vi "MIU_Control_v1.0 (2).vi"() -> ()   [LabVIEW 2010]
uses:
  <vilib>/Instr/_visa.llb/VISA Configure Serial Port (Instr).vi
  <vilib>/Analysis/NI_AALPro.lvlib
panel:
  in  "Tab Control":T1(tab)
  in  "Intrument Serial Input":refnum<visa-resource-name>="COM4"
  in  "data bits":u16=8 min=5 max=8 step=1
  in  "parity":u16(ring) items=["None", "Odd", "Even", "Mark", "Space"]
  in  "stop bits":u16(ring)=10 items=["1.0"=10, "1.5"=15, "2.0"=20]
  in  "flow control":u16(ring) items=["None"=0, "XON/XOFF"=1, "RTS/CTS"=2, "DTR/DSR"=4]
  in  "delay before read (ms)":u32=500
  in  "byte count":u32=500
  out "Incoming Serial String":string
  out "Time":string
  out "Date":string
  in  "stop":bool
  in  "Control Unit Port":refnum<visa-resource-name>="COM4"
  in  "baud rate (9600)":u32=9600
  in  "baud rate (9600)":u32=9600
  out "N2O is FLAT":bool
  out "Rolling CO Slope Fit":cluster{i32[], "Best Linear Fit":dbl[]}[](graph)
  out "CO":dbl(graph)=0.310407
  out "N2O":dbl(graph)
  out "H2O":dbl(graph)
  out "CO PPM":string
  out "N2O PPM":string
  out "H2O PPM":string
  out "CO DRY":dbl(graph)
  out "CO DRY":string
  out "N2O DRY 2":string
  out "N2O DRY":dbl(graph)
  in  "Average Points":i32
  out "slope":dbl
  out "Rolling N2O Slope Fit 2":cluster{i32[], "Best Linear Fit":dbl[]}[](graph)
  out "slope 2":dbl
  in  "N2O Low Limit":dbl
  in  "CO High Limit":dbl
  out "CO is FLAT":bool
  in  "CO Low Limit":dbl
  in  "N2O High Limit":dbl
  out "CELL TEMP":string
  out "CELL TEMPERATURE":dbl(graph)
  out "AMBIENT TEMPERATURE":dbl(graph)
  out "AMBIENT TEMP":string
  out "AIN5":dbl(graph)
  out "SUPERCOOL TEMP":string
  out "LINE LOCK":dbl(graph)
  out "LINELOCK - LASER CONTROL VOLTAGE":string
  out "PRESSURE":dbl(graph)
  out "PRESSURE 2":string
  out "SuperCool Temperature":dbl
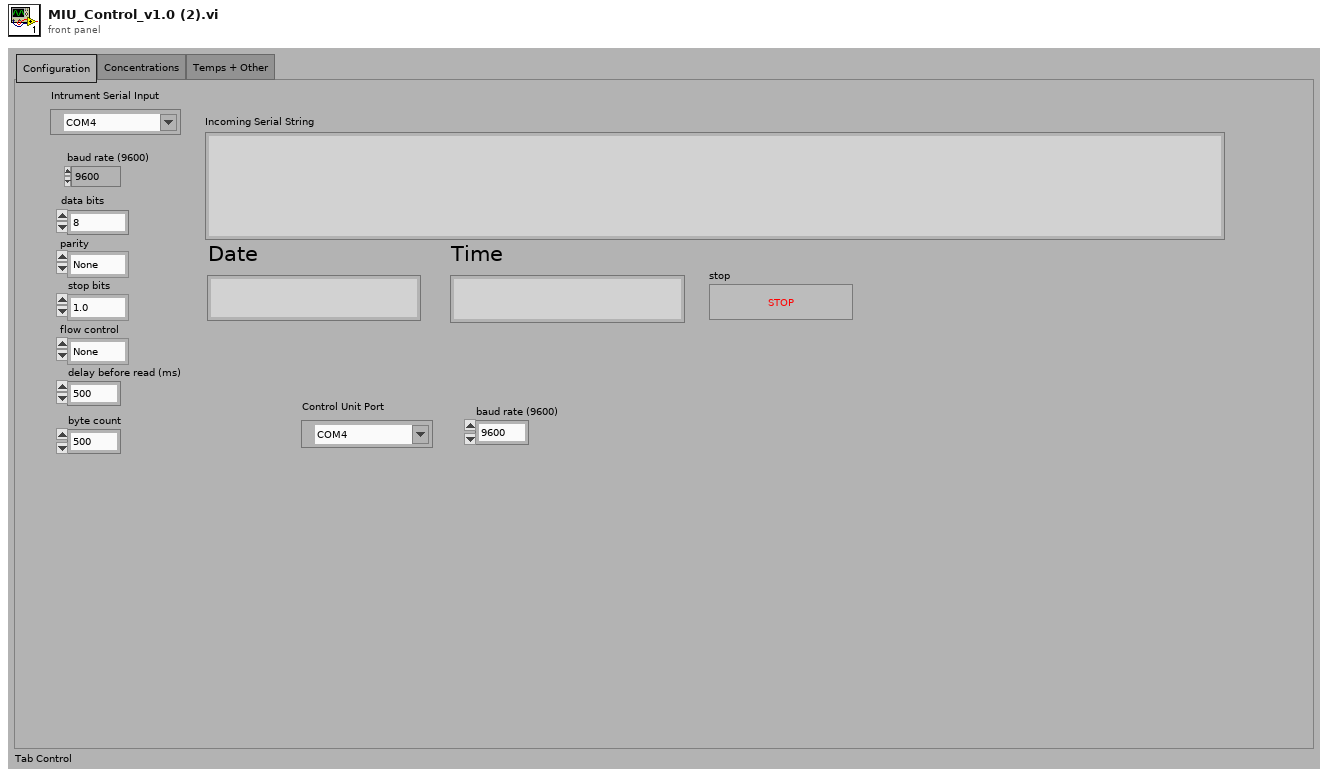
[diagram p1: front panel]
types:
  T1 = enum32{"Configuration", "Concentrations", "Temps + Other"}
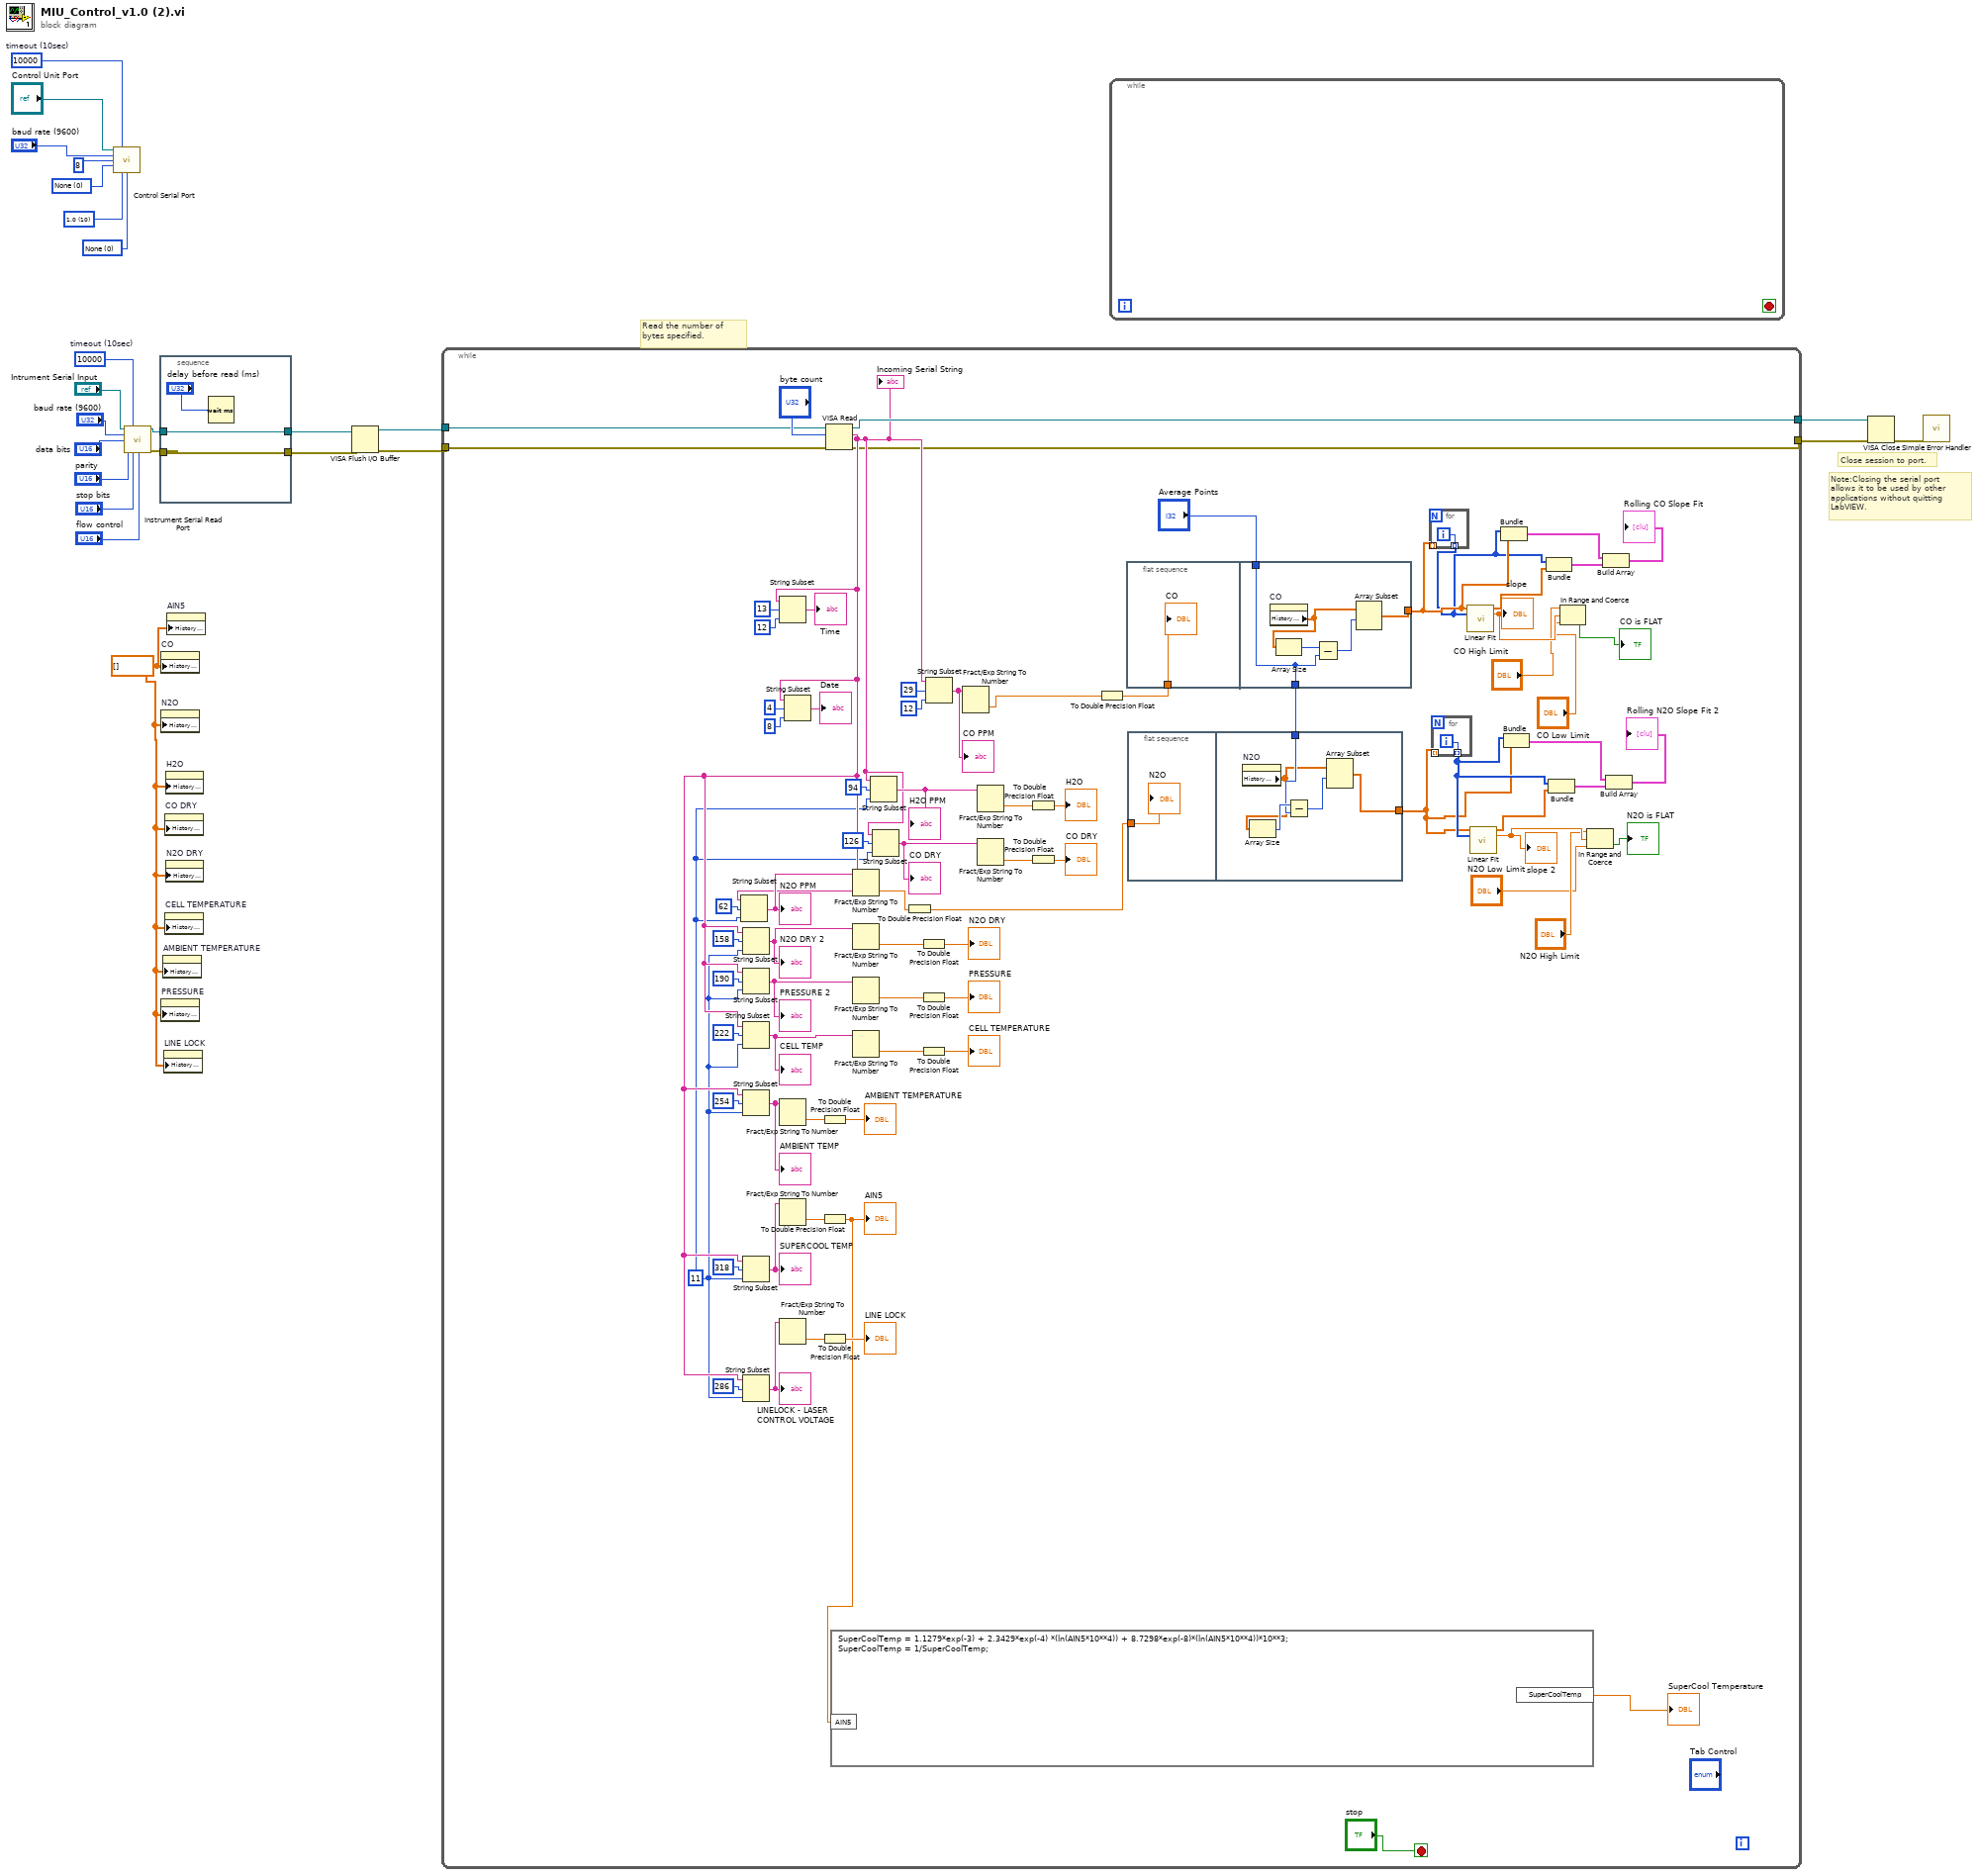
[diagram p0: block diagram]
diagram:
  w3 = u16 0 items=["None"=0, "XON/XOFF"=1, "RTS/CTS"=2, "DTR/DSR"=4] ("flow control")
  w4 = u16 10 items=["1.0"=10, "1.5"=15, "2.0"=20] ("stop bits")
  w6 = u16 0 items=["None", "Odd", "Even", "Mark", "Space"] ("parity")
  w5 = u32 10000  # timeout (10sec)
  w9 = dbl[] [] ("History Data")
  w21 = u32 10000  # timeout (10sec)
  # "Read the number of bytes specified."
  # "Note:Closing the serial port allows it to be used by other applications without quitting LabVIEW."
  # "Close session to port."
  n1 = call-poly "Control Serial Port"("VISA resource name"="Control Unit Port", "timeout (10sec)"=w5, "baud rate (9600)"="baud rate (9600)", "data bits (8)"=u16 8 ("data bits"), "parity (0:none)"=w6, "stop bits (10: 1 bit)"=w4, "flow control (0:none)"=w3) -> ()  [unwired: 2 in, 7 out]
  n2 = call-poly "Instrument Serial Read Port"("VISA resource name"="Intrument Serial Input", "timeout (10sec)"=w21, "baud rate (9600)"="baud rate (9600)", "data bits (8)"="data bits", "parity (0:none)"="parity", "stop bits (10: 1 bit)"="stop bits", "flow control (0:none)"="flow control") -> ("VISA resource name out"=w16:refnum<visa-resource-name>, "error out"=w17:errorcluster)  [unwired: 2 in, 5 out]
  n3 = stacked-sequence {
    tunnel: w17 -> [w27]
    tunnel: [w27] -> w10
    tunnel: w16 -> [w26]
    tunnel: [w26] -> w11
    frame #0 {
      n4 = Wait (ms)(milliseconds to wait="delay before read (ms)") -> ()  [unwired: 1 out]
    }
  }
  n5 = property on="CO" class="WFChart (strict)"("History Data"=w9) -> ()  [unwired: 2 in, 2 out]
  n6 = property on="N2O" class="WFChart (strict)"("History Data"=w9) -> ()  [unwired: 2 in, 2 out]
  n7 = property on="PRESSURE" class="WFChart (strict)"("History Data"=w9) -> ()  [unwired: 2 in, 2 out]
  n8 = property on="AMBIENT TEMPERATURE" class="WFChart (strict)"("History Data"=w9) -> ()  [unwired: 2 in, 2 out]
  n9 = property on="LINE LOCK" class="WFChart (strict)"("History Data"=w9) -> ()  [unwired: 2 in, 2 out]
  n10 = property on="CO DRY" class="WFChart (strict)"("History Data"=w9) -> ()  [unwired: 2 in, 2 out]
  n11 = property on="CELL TEMPERATURE" class="WFChart (strict)"("History Data"=w9) -> ()  [unwired: 2 in, 2 out]
  n12 = property on="H2O" class="WFChart (strict)"("History Data"=w9) -> ()  [unwired: 2 in, 2 out]
  n13 = property on="N2O DRY" class="WFChart (strict)"("History Data"=w9) -> ()  [unwired: 2 in, 2 out]
  n14 = property on="AIN5" class="WFChart (strict)"("History Data"=w9) -> ()  [unwired: 2 in, 2 out]
  n15 = VISA Flush I/O Buffer(VISA resource name=w11, error in (no error)=w10) -> (VISA resource name out=w13:refnum<visa-resource-name>, error out=w12:errorcluster)  [unwired: 1 in]
  n16 = while {
    tunnel: w13 -> [w74]
    tunnel: w12 -> [w75]
    tunnel: [w98] -> w15
    tunnel: [w53] -> w14
    stop <- "stop" stop-if-true
    w64 = 11 ("offset (0)")
    n17 = VISA Read(VISA resource name=w74, byte count="byte count", error in (no error)=w75) -> (VISA resource name out=w98:refnum<visa-resource-name>, read buffer=w65:string, error out=w53:errorcluster)  [unwired: 1 out]
    "Incoming Serial String" <- w65
    n18 = String Subset(string=w65, offset (0)=62, length (rest)=w64) -> (substring=w91:string)
    "N2O PPM" <- w91
    n19 = String Subset(string=w65, offset (0)=158, length (rest)=w64) -> (substring=w78:string)
    "N2O DRY 2" <- w78
    n20 = String Subset(string=w65, offset (0)=190, length (rest)=w64) -> (substring=w77:string)
    "PRESSURE 2" <- w77
    n21 = String Subset(string=w65, offset (0)=222, length (rest)=w64) -> (substring=w76:string)
    "CELL TEMP" <- w76
    n22 = String Subset(string=w65, offset (0)=254, length (rest)=w64) -> (substring=w68:string)
    "AMBIENT TEMP" <- w68
    n23 = String Subset(string=w65, offset (0)=318, length (rest)=w64) -> (substring=w66:string)
    "SUPERCOOL TEMP" <- w66
    n24 = String Subset(string=w65, offset (0)=286, length (rest)=w64) -> (substring=w67:string)
    "LINELOCK - LASER CONTROL VOLTAGE" <- w67
    n25 = String Subset(string=w65, offset (0)=13, length (rest)=12 ("length (rest)")) -> (substring=→"Time":string)
    n26 = Fract/Exp String To Number(string=w68) -> (number=w72:dbl)  [unwired: 3 in, 1 out]
    n27 = Fract/Exp String To Number(string=w66) -> (number=w69:dbl)  [unwired: 3 in, 1 out]
    n28 = Fract/Exp String To Number(string=w67) -> (number=w70:dbl)  [unwired: 3 in, 1 out]
    n29 = String Subset(string=w65, offset (0)=4, length (rest)=8 ("length (rest)")) -> (substring=→"Date":string)
    n30 = To Double Precision Float(number=w72) -> (double precision float=→"AMBIENT TEMPERATURE":dbl)
    n31 = To Double Precision Float(number=w69) -> (double precision float=w55:dbl)
    "AIN5" <- w55
    n32 = To Double Precision Float(number=w70) -> (double precision float=→"LINE LOCK":dbl)
    n33 = formula code="SuperCoolTemp = 1.1279*exp(-3) + 2.3429*exp(-4) *(ln(AIN5*10**4)) + 8.7298*exp(-8)*(ln(AIN5*10**4))*10**3;\nSuperCoolTemp = 1/SuperCoolTemp;"("AIN5"=w55) -> ("SuperCoolTemp"=→"SuperCool Temperature":dbl)
    n34 = Fract/Exp String To Number(string=w91) -> (number=w45:dbl)  [unwired: 3 in, 1 out]
    n35 = Fract/Exp String To Number(string=w78) -> (number=w84:dbl)  [unwired: 3 in, 1 out]
    n36 = Fract/Exp String To Number(string=w77) -> (number=w82:dbl)  [unwired: 3 in, 1 out]
    n37 = Fract/Exp String To Number(string=w76) -> (number=w80:dbl)  [unwired: 3 in, 1 out]
    n38 = String Subset(string=w65, offset (0)=94, length (rest)=w64) -> (substring=w90:string)
    "H2O PPM" <- w90
    n39 = String Subset(string=w65, offset (0)=126, length (rest)=w64) -> (substring=w79:string)
    "CO DRY" <- w79
    n40 = To Double Precision Float(number=w45) -> (double precision float=w44:dbl)
    n41 = To Double Precision Float(number=w84) -> (double precision float=→"N2O DRY":dbl)
    n42 = To Double Precision Float(number=w82) -> (double precision float=→"PRESSURE":dbl)
    n43 = To Double Precision Float(number=w80) -> (double precision float=→"CELL TEMPERATURE":dbl)
    n44 = String Subset(string=w65, offset (0)=29, length (rest)=12 ("length (rest)")) -> (substring=w92:string)
    "CO PPM" <- w92
    n45 = Fract/Exp String To Number(string=w92) -> (number=w89:dbl)  [unwired: 3 in, 1 out]
    n46 = Fract/Exp String To Number(string=w90) -> (number=w88:dbl)  [unwired: 3 in, 1 out]
    n47 = Fract/Exp String To Number(string=w79) -> (number=w86:dbl)  [unwired: 3 in, 1 out]
    n48 = To Double Precision Float(number=w88) -> (double precision float=→"H2O":dbl)
    n49 = To Double Precision Float(number=w86) -> (double precision float=→"CO DRY":dbl)
    n50 = To Double Precision Float(number=w89) -> (double precision float=w52:dbl)
    n51 = flat-sequence {
      tunnel: w52 -> [w114]
      tunnel: [w116] -> w51
      tunnel: "Average Points" -> [w115]
      tunnel: [w115] -> w42
      frame #0 {
        "CO" <- w114
      }
      frame #1 {
        n52 = property on="CO" class="WFChart (strict)"() -> ("History Data"=w117:dbl[])  [unwired: 2 in, 2 out]
        n53 = Array Size(array=w117) -> (size(s)=w118:i32)
        n54 = Subtract(x=w118, y=w115) -> (x-y=w119:i32)
        n55 = Array Subset(array=w117, index=w119) -> (w116:dbl[])  [unwired: 1 in]
      }
    }
    n56 = flat-sequence {
      tunnel: w44 -> [w107]
      tunnel: w42 -> [w110]
      tunnel: [w108] -> w36
      frame #0 {
        "N2O" <- w107
      }
      frame #1 {
        n57 = property on="N2O" class="WFChart (strict)"() -> ("History Data"=w109:dbl[])  [unwired: 2 in, 2 out]
        n58 = Array Size(array=w109) -> (size(s)=w111:i32)
        n59 = Subtract(x=w111, y=w110) -> (x-y=w112:i32)
        n60 = Array Subset(array=w109, index=w112) -> (w108:dbl[])  [unwired: 1 in]
      }
    }
    n61 = for {
      tunnel: [w113] -> w50 mode=indexing
      tunnel: w51 -> [_] mode=indexing
      i -> [w113]
    }
    n62 = for {
      tunnel: [w106] -> w41 mode=indexing
      tunnel: w36 -> [_] mode=indexing
      i -> [w106]
    }
    n63 = call <vilib>:"Linear Fit.vi"("Y"=w51, "X"=w50) -> ("Best Linear Fit"=w49:dbl[], "slope"=w35:dbl)  [unwired: 9 in, 3 out]
    "slope" <- w35
    n64 = call <vilib>:"Linear Fit.vi"("Y"=w36, "X"=w41) -> ("Best Linear Fit"=w40:dbl[], "slope"=w30:dbl)  [unwired: 9 in, 3 out]
    "slope 2" <- w30
    n65 = Bundle(w50, w51) -> (w48:cluster{i32[], dbl[]})  [unwired: 1 in]
    n66 = Bundle(w41, w36) -> (w39:cluster{i32[], dbl[]})  [unwired: 1 in]
    n67 = Bundle(w50, "Best Linear Fit"=w49) -> (w47:cluster{i32[], "Best Linear Fit":dbl[]})  [unwired: 1 in]
    n68 = Bundle(w41, "Best Linear Fit"=w40) -> (w38:cluster{i32[], "Best Linear Fit":dbl[]})  [unwired: 1 in]
    n69 = In Range and Coerce(upper limit="CO High Limit", x=w35, lower limit="CO Low Limit") -> (In Range?=→"CO is FLAT":bool)  [unwired: 1 out]
    n70 = In Range and Coerce(upper limit="N2O High Limit", x=w30, lower limit="N2O Low Limit") -> (In Range?=→"N2O is FLAT":bool)  [unwired: 1 out]
    n71 = Build Array(w48, w47) -> (→"Rolling CO Slope Fit":cluster{i32[], "Best Linear Fit":dbl[]}[])
    n72 = Build Array(w39, w38) -> (→"Rolling N2O Slope Fit 2":cluster{i32[], "Best Linear Fit":dbl[]}[])
  }
  n73 = while {
    stop <- _ stop-if-true
  }
  n74 = VISA Close(VISA resource name=w15, error in (no error)=w14) -> (error out=w23:errorcluster)
  n75 = call <vilib>:"Simple Error Handler.vi"("error in (no error)"=w23) -> ()  [unwired: 1 in, 8 out]
